vi "测量流程.vi"(11 "控制命令":T1(ring)) -> ()   [LabVIEW 2016, in "斯坦道CODcr.lvlib"]
uses:
  <vilib>/ptbypt/NI_PtbyPt.lvlib
panel:
  out "记录运行时间":timestamp
  out "start":timestamp
  out "重测":bool
  out "x-y":dbl
  out "当前时间":timestamp
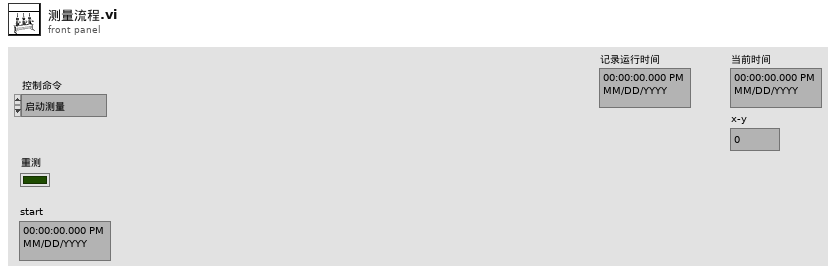
[diagram p1: front panel]
types:
  T1 = enum16{"启动测量", "标样核查", "零点核查", "跨度核查", "空白测试", "平行样测试", "加标回收", "空白校准", "标样校准", "初始化（清洗）", "停止测试", "仪器重启", "校时", "模式设置", "测量间隔设置"}
  T2 = cluster{"站号":u16, "量程切换":enum32{"H", "L", "AUTO"}, "控制命令":enum16{"启动测量", "标样核查", "零点核查", "跨度核查", "空白测试", "平行样测试", "加标回收", "空白校准", "标样校准", "初始化（清洗）", "停止测试", "仪器重启", "校时", "模式设置", "测量间隔设置"}, "模式设置":enum16{"待机", "连续模式", "周期模式", "定点模式", "受控模式", "手动模式"}, "测量间隔":u16}
  T3 = typedef "报警信息字段定义.ctl" = cluster{"时间":timestamp, "参数":string, "元器件":string, "故障现象":string, "故障分析":string, "state":string, "code":string, "platform_alarm_code":string}
  T4 = cluster{"时间标识":timestamp, "设备":string, "日志信息":string, "流程参数":string}
  T5 = enum16{"空闲", "水样测试", "标样核查", "零点核查", "跨度核查", "空白测试", "平行样测试", "加标回收", "空白校准", "标样校准", "初始化（清洗）"}
  T6 = cluster{"系统时间":timestamp, "工作状态":u16, "测量模式":enum16{"待机", "连续模式", "周期模式", "定点模式", "受控模式", "手动模式"}, "告警代码":u16, "故障代码":u16, "日志代码":u16, "软件版本":u16, "F0":sgl, "F1":sgl, "F2":sgl, "F3":sgl, "T":sgl, "H":sgl, "id":u16, "flowid":u16, "量程":u16, "总磷控温温度1":sgl, "营养盐控温温度2":sgl, "ADC":sgl}
  T7 = cluster{"水样测试量程模式":enum16{"H", "L", "AUTO"}, "空白核查量程模式":enum16{"H", "L", "AUTO"}, "跨度核查量程模式":enum16{"H", "L", "AUTO"}, "加标回收量程模式":enum16{"H", "L", "AUTO"}, "标样核查量程模式":enum16{"H", "L", "AUTO"}}
  T8 = cluster{"因子编码":u32, "单位":u16, "标样参考值":sgl, "水样数据时间":timestamp, "水样实测值":sgl, "水样数据标识":string, "标样数据时间":timestamp, "标样实测值":sgl, "标样数据标识":string, "空白数据时间":timestamp, "空白实测值":sgl, "空白数据标识":string, "零点核查数据时间":timestamp, "零点核查实测值":sgl, "零点核查数据标识":string, "跨度核查数据时间":timestamp, "跨度核查实测值":sgl, "跨度核查数据标识":string, "加标回收数据时间":timestamp, "加标回收实测值":sgl, "加标回收数据标识":string, "平行样数据时间":timestamp, "平行样实测值":sgl, "平行样数据标识":string, "F0":sgl, "F1":sgl, "F2":sgl, "F3":sgl, "F4":sgl, "F5":sgl, "F6":sgl, "F7":sgl, "温度":sgl, "湿度":sgl, "X值":sgl, "fidrange":u16, "X1值":sgl}[]
  T9 = cluster{"因子编码":u32, "单位":u16, "标样参考值":sgl, "水样数据时间":timestamp, "水样实测值":sgl, "水样数据标识":string, "标样数据时间":timestamp, "标样实测值":sgl, "标样数据标识":string, "空白数据时间":timestamp, "空白实测值":sgl, "空白数据标识":string, "零点核查数据时间":timestamp, "零点核查实测值":sgl, "零点核查数据标识":string, "跨度核查数据时间":timestamp, "跨度核查实测值":sgl, "跨度核查数据标识":string, "加标回收数据时间":timestamp, "加标回收实测值":sgl, "加标回收数据标识":string, "平行样数据时间":timestamp, "平行样实测值":sgl, "平行样数据标识":string, "F0":sgl, "F1":sgl, "F2":sgl, "F3":sgl, "F4":sgl, "F5":sgl, "F6":sgl, "F7":sgl, "温度":sgl, "湿度":sgl, "X值":sgl, "fidrange":u16, "X1值":sgl}
  T10 = cluster{"总磷跨度值":dbl, "总磷零点标准液浓度":dbl, "总磷跨度标准液浓度":dbl, "总磷标准液标准浓度":dbl, "总氮跨度值":dbl, "总氮零点标准液浓度":dbl, "总氮跨度标准液浓度":dbl, "总氮标准液标准浓度":dbl, "COD跨度值":dbl, "COD零点标准液浓度":dbl, "COD跨度标准液浓度":dbl, "COD标准液标准浓度":dbl, "氨氮跨度值":dbl, "氨氮零点标准液浓度":dbl, "氨氮跨度标准液浓度":dbl, "氨氮标准液标准浓度":dbl, "磷酸盐跨度值":dbl, "磷酸盐零点标准液浓度":dbl, "磷酸盐跨度标准液浓度":dbl, "磷酸盐标准液标准浓度":dbl, "硝氮跨度值":dbl, "硝氮零点标准液浓度":dbl, "硝氮跨度标准液浓度":dbl, "硝氮标准液标准浓度":dbl, "亚硝氮跨度值":dbl, "亚硝氮零点标准液浓度":dbl, "亚硝氮跨度标准液浓度":dbl, "亚硝氮标准液标准浓度":dbl, "硫化物跨度值":dbl, "硫化物零点标准液浓度":dbl, "硫化物跨度标准液浓度":dbl, "硫化物标准液标准浓度":dbl, "硅酸盐跨度值":dbl, "硅酸盐零点标准液浓度":dbl, "硅酸盐跨度标准液浓度":dbl, "硅酸盐标准液标准浓度":dbl, "总磷零点标准液偏差":dbl, "总磷跨度标准液偏差":dbl, "总磷标准液标准偏差":dbl, "总氮零点标准液偏差":dbl, "总氮跨度标准液偏差":dbl, "总氮标准液标准偏差":dbl, "COD零点标准液偏差":dbl, "COD跨度标准液偏差":dbl, "COD标准液标准偏差":dbl, "氨氮零点标准液偏差":dbl, "氨氮跨度标准液偏差":dbl, "氨氮标准液标准偏差":dbl, "磷酸盐零点标准液偏差":dbl, "磷酸盐跨度标准液偏差":dbl, "磷酸盐标准液标准偏差":dbl, "硝氮零点标准液偏差":dbl, "硝氮跨度标准液偏差":dbl, "硝氮标准液标准偏差":dbl, "亚硝氮零点标准液偏差":dbl, "亚硝氮跨度标准液偏差":dbl, "亚硝氮标准液标准偏差":dbl, "硫化物零点标准液偏差":dbl, "硫化物跨度标准液偏差":dbl, "硫化物标准液标准偏差":dbl, "硅酸盐零点标准液偏差":dbl, "硅酸盐跨度标准液偏差":dbl, "硅酸盐标准液标准偏差":dbl, "氟化物跨度值":dbl, "氟化物零点标准液浓度":dbl, "氟化物跨度标准液浓度":dbl, "氟化物标准液标准浓度":dbl, "氟化物零点标准液偏差":dbl, "氟化物跨度标准液偏差":dbl, "氟化物标准液标准偏差":dbl, "CODMn跨度值":dbl, "CODMn零点标准液浓度":dbl, "CODMn跨度标准液浓度":dbl, "CODMn标准液标准浓度":dbl, "CODMn零点标准液偏差":dbl, "CODMn跨度标准液偏差":dbl, "CODMn标准液标准偏差":dbl}
  T11 = typedef "LVDateTimeRec.ctl" = cluster{"秒数的小数部分":dbl, "秒":i32, "分":i32, "时":i32, "日":i32, "月":i32, "年":i32, "天数（周）":i32, "天数（年）":i32, "DST":i32}
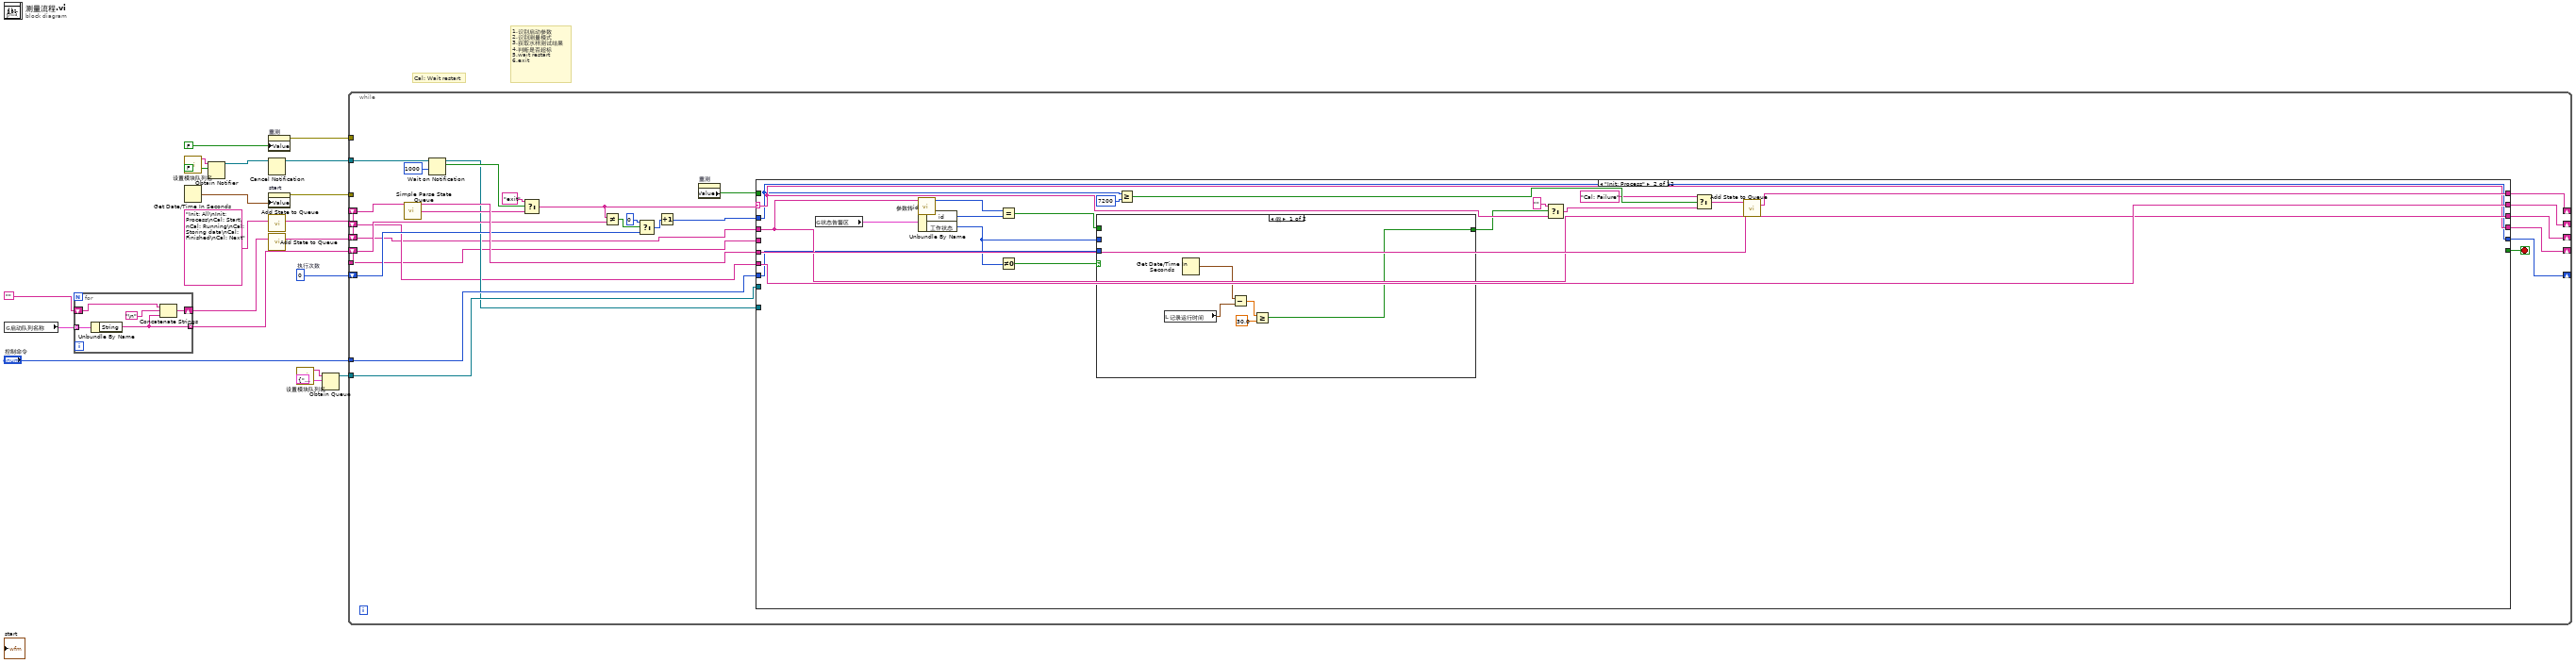
[diagram p0: block diagram]
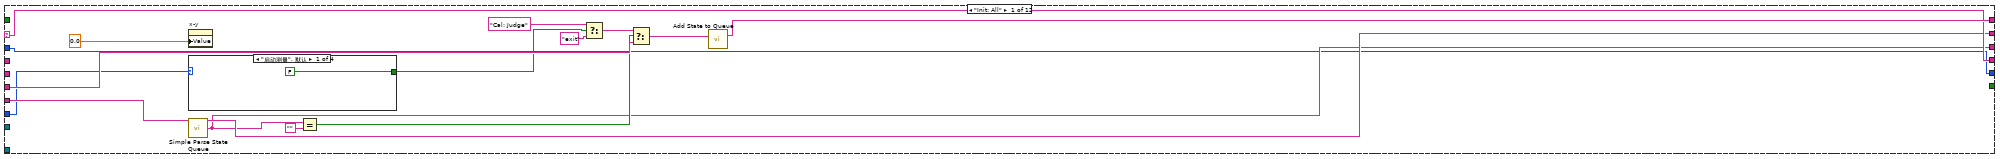
[diagram p2: hidden frame]
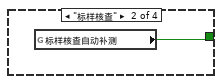
[diagram p3: hidden frame]
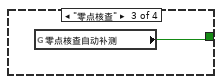
[diagram p4: hidden frame]
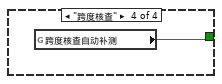
[diagram p5: hidden frame]
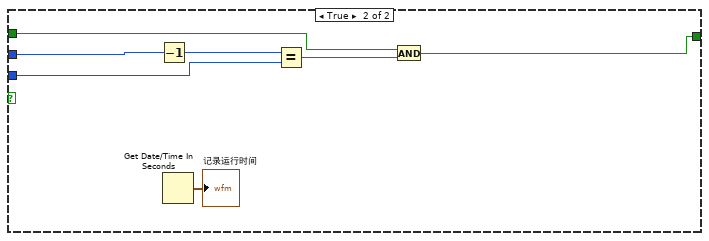
[diagram p6: hidden frame]
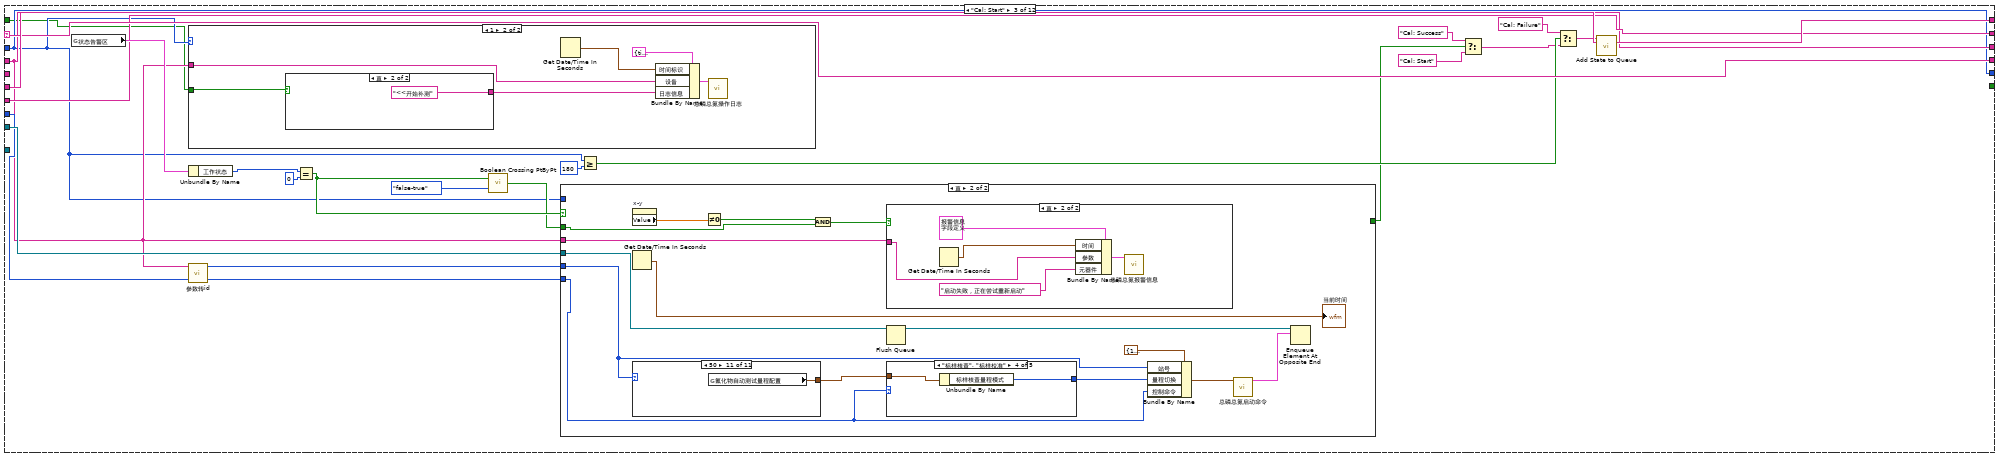
[diagram p7: hidden frame]
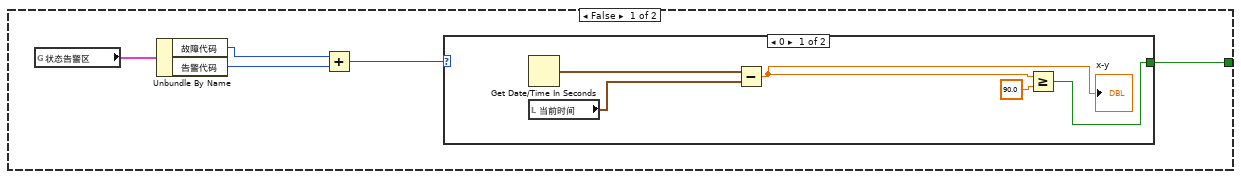
[diagram p8: hidden frame]
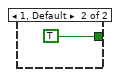
[diagram p9: hidden frame]
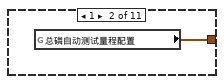
[diagram p12: hidden frame]
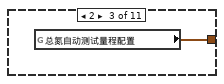
[diagram p13: hidden frame]
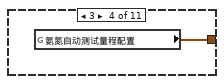
[diagram p14: hidden frame]
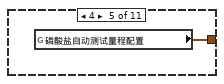
[diagram p15: hidden frame]
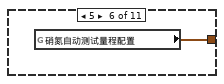
[diagram p16: hidden frame]
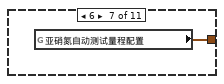
[diagram p17: hidden frame]
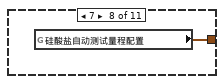
[diagram p18: hidden frame]
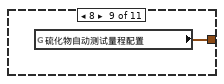
[diagram p19: hidden frame]
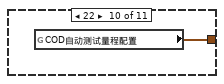
[diagram p20: hidden frame]
diagram:
  w14 = 0  # 执行次数
  # "Cal: Wait restart"
  # "1.识别启动参数\n2.识别测量模式\n3.获取水样测试结果\n4.判断是否超标\n5.wait restart\n6.exit"
  n1 = global read "model config var.vi" "启动队列名称"() -> (w7:cluster{"String":string, "Value":u16}[])
  n2 = for {
    shift-right: [w24] -> w8
    shift-left: "" -> [w25]
    tunnel: w7 -> [w23] mode=indexing
    tunnel: [w21] -> w1 mode=indexing
    n3 = Unbundle By Name(w23) -> ("String"=w21:string)
    n4 = Concatenate Strings(w25, "\n", w21) -> (w24:string)
  }
  n5 = call "设置模块队列名.vi"() -> ("Msg"=w12:string)  [unwired: 5 in]
  n6 = Get Date/Time In Seconds() -> (seconds since 1Jan1904=w2:timestamp)
  n7 = Obtain Notifier(name (unnamed)=w12, notification data type=FALSE) -> (notifier out=w19:refnum<notifier>)  [unwired: 2 in, 2 out]
  n8 = property on="重测" class="Bool (严格)"("Value"=FALSE ("重测")) -> (error out=w4:errorcluster)  [unwired: 2 in, 1 out]
  n9 = Cancel Notification(0:w19) -> (8:w10:refnum<notifier>)  [unwired: 1 in, 2 out]
  n10 = property on="start" class="AbsTime (严格)"("Value"=w2) -> (error out=w3:errorcluster)  [unwired: 2 in, 1 out]
  n11 = call "Add State to Queue.vi"("State(s) In (\"\")"="Init: All\nInit: Process\nCal: Start\nCal: Running\nCal: Storing data\nCal: Finished\nCal: Next" ("State(s) In (\"\")")) -> ("States Out"=w17:string)  [unwired: 14 in]
  n12 = call "Add State to Queue.vi"("State(s) In (\"\")"=w8) -> ("States Out"=w13:string)  [unwired: 14 in]
  n13 = call "设置模块队列名.vi"() -> ("Msg"=w11:string)  [unwired: 5 in]
  n14 = Obtain Queue(name (unnamed)=w11, element data type=cluster{"命令":string, "data":variant} {"命令"="", "data"=variant}) -> (queue out=w15:refnum<queue>)  [unwired: 3 in, 2 out]
  n15 = while {
    tunnel: w15 -> [w50]
    shift-right: [w49] -> _
    shift-left: w17 -> [w52]
    shift-right: [w43] -> _
    shift-left: w14 -> [w46]
    shift-right: [w27] -> _
    shift-left: _ -> [w48]
    tunnel: "控制命令" -> [w41]
    shift-right: [w39] -> _
    shift-left: w13 -> [w30]
    shift-right: [w28] -> _
    shift-left: _ -> [w29]
    tunnel: w10 -> [w37]
    tunnel: w4 -> [_]
    tunnel: w3 -> [_]
    tunnel: w1 -> [w26]
    stop <- w40 stop-if-true
    n16 = call "Simple Parse State Queue.vi"("State Queue"=w52) -> ("Remain States"=w51:string, "Next State"=w34:string)  [unwired: 13 in]
    n17 = Wait on Notification(notifier=w37, timeout in ms (-1)=1000 ("超时毫秒(-1)")) -> (notifier out=w32:refnum<notifier>, notification=w36:bool)  [unwired: 2 in, 2 out]
    n18 = Select(t="exit", s=w36, f=w34) -> (s? t:f=w33:string)
    n19 = Not Equal?(x=w33, y=w48) -> (x != y?=w47:bool)
    n20 = Select(t=0, s=w47, f=w46) -> (s? t:f=w44:i32)
    n21 = Increment(x=w44) -> (x+1=w42:i32)
    n22 = property on="重测" class="Bool (严格)"() -> ("Value"=w31:bool)  [unwired: 2 in, 2 out]
    n23 = case shown="\"Init: Process\"" w33 {
      selector: w33 -> [w67 w81 w126 w191 w206 w212 w226 w243 w260 w273 w437 w458]
      tunnel: w51 -> [w64 w91 w128 w193 _ w223 w231 w245 w257 _ _ w459]
      tunnel: w50 -> [_ _ w124 _ _ _ _ _ _ _ _ w455]
      tunnel: [w68 w92 w127 w192 w207 w222 w230 w244 w256 w261 w445 w459] -> w49
      tunnel: [w67 w81 w126 w191 w206 w212 w226 w243 w260 w273 w437 w458] -> w27
      tunnel: [w58 w80 w106 w190 w205 w215 w229 w241 w255 w274 w448 w457] -> w43
      tunnel: w42 -> [w58 w80 w106 w190 w205 w215 w229 w241 w255 w274 w448 w457]
      tunnel: w41 -> [w57 w85 w123 _ _ _ _ _ _ w272 _ _]
      tunnel: [_ _ _ _ _ _ _ _ _ _ _ TRUE] -> w40
      tunnel: w30 -> [w62 w90 w114 w189 w199 w209 w233 w242 w259 w267 w447 w456]
      tunnel: [w59 w88 w108 w188 w198 w208 w232 w240 w258 w269 w446 w453] -> w28
      tunnel: [w61 w90 w114 w189 w199 w209 w233 w242 w259 w266 w447 w456] -> w39
      tunnel: w29 -> [_ w88 w108 w188 w198 w208 w232 w240 w258 w269 w446 w453]
      tunnel: w32 -> [_ _ _ _ _ _ _ _ _ _ _ w454]
      tunnel: w31 -> [_ _ w105 _ _ _ _ w239 _ w271 _ _]
      tunnel: w26 -> [_ _ _ _ _ _ _ _ _ w268 _ _]
      frame "Init: All" {
        n24 = property on="x-y" class="DigNum (严格)"("Value"=0.0 ("x-y")) -> ()  [unwired: 2 in, 2 out]
        n25 = case shown="\"启动测量\", 默认" w57 {
          tunnel: [FALSE ("跨度核查自动补测") w70 w71 w72] -> w56
          frame "启动测量", Default {
          }
          frame "标样核查" {
            n26 = global read "总磷总氮断电保存全局变量.vi" "标样核查自动补测"() -> (w70:bool)
          }
          frame "零点核查" {
            n27 = global read "总磷总氮断电保存全局变量.vi" "零点核查自动补测"() -> (w71:bool)
          }
          frame "跨度核查" {
            n28 = global read "总磷总氮断电保存全局变量.vi" "跨度核查自动补测"() -> (w72:bool)
          }
        }
        n29 = call "Simple Parse State Queue.vi"("State Queue"=w62) -> ("Remain States"=w61:string, "Next State"=w59:string)  [unwired: 13 in]
        n30 = Equal?(x=w59, y="") -> (x = y?=w60:bool)
        n31 = Select(t="Cal: Judge", s=w56, f="exit") -> (s? t:f=w53:string)
        n32 = Select(t=w53, s=w60, f=w64) -> (s? t:f=w63:string)
        n33 = call "Add State to Queue.vi"("State(s) In (\"\")"=w63) -> ("States Out"=w68:string)  [unwired: 14 in]
      }
      frame "Init: Process" {
        n34 = global read "VAR总磷总氮全局变量.vi" "状态告警区"() -> (w89:T6)
        n35 = call "参数转id.vi"("table"=w88) -> ("id"=w86:u16)  [unwired: 10 in]
        n36 = Unbundle By Name(w89) -> ("id"=w87:u16, "工作状态"=w83:u16)
        n37 = Equal?(x=w86, y=w87) -> (x = y?=w74:bool)
        n38 = Not Equal To 0?(x=w83) -> (x != 0?=w84:bool)
        n39 = case shown="假" w84 {
          tunnel: w83 -> [_ w104]
          tunnel: w85 -> [_ w102]
          tunnel: [w93 w99] -> w73
          tunnel: w74 -> [_ w100]
          frame False {
            n40 = local read "记录运行时间"() -> (w97:timestamp)
            n41 = Get Date/Time In Seconds() -> (seconds since 1Jan1904=w96:timestamp)
            n42 = Subtract(x=w96, y=w97) -> (x-y=w95:dbl)
            n43 = Greater Or Equal?(x=w95, y=30.0) -> (x >= y?=w93:bool)
          }
          frame True {
            n44 = Decrement(x=w104) -> (x-1=w103:u16)
            n45 = Get Date/Time In Seconds() -> (seconds since 1Jan1904=→"记录运行时间":timestamp)
            n46 = Equal?(x=w103, y=w102) -> (x = y?=w101:bool)
            n47 = And(x=w100, y=w101) -> (x .and. y?=w99:bool)
          }
        }
        n48 = Greater Or Equal?(x=w80, y=7200) -> (x >= y?=w78:bool)
        n49 = Select(t="", s=w73, f=w81) -> (s? t:f=w76:string)
        n50 = Select(t="Cal: Failure", s=w78, f=w76) -> (s? t:f=w75:string)
        n51 = call "Add State to Queue.vi"("State(s) In Front (\"\")"=w75, "State(s) In (\"\")"=w91) -> ("States Out"=w92:string)  [unwired: 13 in]
      }
      frame "Cal: Start" {
        n52 = global read "VAR总磷总氮全局变量.vi" "状态告警区"() -> (w125:T6)
        n53 = case shown="1" w106 {
          tunnel: w108 -> [_ w181]
          tunnel: w105 -> [_ w180]
          frame 0, Default {
          }
          frame 1 {
            n54 = case shown="真" w180 {
              tunnel: ["<<开始测量" ("日志信息") "<<开始补测" ("日志信息")] -> w182
              frame False {
              }
              frame True {
              }
            }
            n55 = Get Date/Time In Seconds() -> (seconds since 1Jan1904=w185:timestamp)
            n56 = Bundle By Name(cluster=T4 {"时间标识"=timestamp(0 s since 1904-01-01), "设备"="", "日志信息"="", "流程参数"=""} ("data in"), "时间标识"=w185, "设备"=w181, "日志信息"=w182) -> (w184:T4)
            n57 = call "总磷总氮操作日志.vi"("data in"=w184) -> ()  [unwired: 10 in, 1 out]
          }
        }
        n58 = Unbundle By Name(w125) -> ("工作状态"=w113:u16)
        n59 = call "参数转id.vi"("table"=w108) -> ("id"=w107:u16)  [unwired: 10 in]
        n60 = Equal?(x=w113, y=u16 0) -> (x = y?=w111:bool)
        n61 = call <vilib>:"Boolean Crossing PtByPt.vi"("direction"=enum16{"either", "false-true", "true-false"}."false-true", "input"=w111) -> ("crossing"=w109:bool)  [unwired: 1 in]
        n62 = case shown="真" w111 {
          tunnel: w123 -> [_ w150]
          tunnel: w124 -> [_ w153]
          tunnel: [w133 _] -> w118
          tunnel: w107 -> [_ w148]
          tunnel: w106 -> [_ _]
          tunnel: w108 -> [_ w142]
          tunnel: w109 -> [_ w140]
          frame False {
            n63 = global read "VAR总磷总氮全局变量.vi" "状态告警区"() -> (w132:T6)
            n64 = Unbundle By Name(w132) -> ("故障代码"=w130:u16, "告警代码"=w131:u16)
            n65 = Add(x=w130, y=w131) -> (x+y=w129:u16)
            n66 = case shown="0" w129 {
              tunnel: [w134 TRUE] -> w133
              frame 0 {
                n67 = Get Date/Time In Seconds() -> (seconds since 1Jan1904=w137:timestamp)
                n68 = local read "当前时间"() -> (w138:timestamp)
                n69 = Subtract(x=w137, y=w138) -> (x-y=w136:dbl)
                "x-y" <- w136
                n70 = Greater Or Equal?(x=w136, y=90.0) -> (x >= y?=w134:bool)
              }
              frame 1, Default {
              }
            }
          }
          frame True {
            n71 = property on="x-y" class="DigNum (严格)"() -> ("Value"=w144:dbl)  [unwired: 2 in, 2 out]
            n72 = Get Date/Time In Seconds() -> (seconds since 1Jan1904=→"当前时间":timestamp)
            n73 = case shown="50" w148 {
              tunnel: [_ w160 w161 w162 w163 w164 w165 w166 w167 w168 w169] -> w149
              frame 0, Default {
              }
              frame 1 {
                n74 = global read "总磷总氮断电保存全局变量.vi" "总磷自动测试量程配置"() -> (w160:T7)
              }
              frame 2 {
                n75 = global read "总磷总氮断电保存全局变量.vi" "总氮自动测试量程配置"() -> (w161:T7)
              }
              frame 3 {
                n76 = global read "总磷总氮断电保存全局变量.vi" "氨氮自动测试量程配置"() -> (w162:T7)
              }
              frame 4 {
                n77 = global read "总磷总氮断电保存全局变量.vi" "磷酸盐自动测试量程配置"() -> (w163:T7)
              }
              frame 5 {
                n78 = global read "总磷总氮断电保存全局变量.vi" "硝氮自动测试量程配置"() -> (w164:T7)
              }
              frame 6 {
                n79 = global read "总磷总氮断电保存全局变量.vi" "亚硝氮自动测试量程配置"() -> (w165:T7)
              }
              frame 7 {
                n80 = global read "总磷总氮断电保存全局变量.vi" "硅酸盐自动测试量程配置"() -> (w166:T7)
              }
              frame 8 {
                n81 = global read "总磷总氮断电保存全局变量.vi" "硫化物自动测试量程配置"() -> (w167:T7)
              }
              frame 22 {
                n82 = global read "总磷总氮断电保存全局变量.vi" "COD自动测试量程配置"() -> (w168:T7)
              }
              frame 50 {
                n83 = global read "总磷总氮断电保存全局变量.vi" "氟化物自动测试量程配置"() -> (w169:T7)
              }
            }
            n84 = Not Equal To 0?(x=w144) -> (x != 0?=w143:bool)
            n85 = And(x=w143, y=w140) -> (x .and. y?=w141:bool)
            n86 = case shown="真" w141 {
              tunnel: w142 -> [_ w157]
              frame False {
              }
              frame True {
                n87 = Get Date/Time In Seconds() -> (seconds since 1Jan1904=w156:timestamp)
                n88 = Bundle By Name(cluster=T3 {"时间"=timestamp(0 s since 1904-01-01), "参数"="", "元器件"="", "故障现象"="", "故障分析"="", "state"="", "code"="", "platform_alarm_code"=""} ("data in"), "时间"=w156, "参数"=w157, "元器件"="启动失败，正在尝试重新启动" ("报警信息")) -> (w158:T3)
                n89 = call "总磷总氮报警信息.vi"("data in"=w158) -> ()  [unwired: 10 in, 1 out]
              }
            }
            n90 = Flush Queue(queue=w153) -> (queue out=w146:refnum<queue>)  [unwired: 1 in, 2 out]
            n91 = case shown="\"标样核查\", \"标样校准\"" w150 {
              tunnel: w149 -> [w171 w173 w175 w177 w179]
              tunnel: [w170 w172 w174 w176 w178] -> w154
              frame "启动测量", Default {
                n92 = Unbundle By Name(w171) -> ("水样测试量程模式"=w170:enum16{"H", "L", "AUTO"})
              }
              frame "零点核查", "空白测试", "空白校准" {
                n93 = Unbundle By Name(w173) -> ("空白核查量程模式"=w172:enum16{"H", "L", "AUTO"})
              }
              frame "跨度核查" {
                n94 = Unbundle By Name(w175) -> ("跨度核查量程模式"=w174:enum16{"H", "L", "AUTO"})
              }
              frame "标样核查", "标样校准" {
                n95 = Unbundle By Name(w177) -> ("标样核查量程模式"=w176:enum16{"H", "L", "AUTO"})
              }
              frame "加标回收" {
                n96 = Unbundle By Name(w179) -> ("加标回收量程模式"=w178:enum16{"H", "L", "AUTO"})
              }
            }
            n97 = Bundle By Name(cluster=T2 {"站号"=1, "量程切换"=enum."AUTO", "控制命令"=enum."启动测量", "模式设置"=enum."待机", "测量间隔"=0} ("参数"), "站号"=w148, "量程切换"=w154, "控制命令"=w150) -> (w151:T2)
            n98 = call "总磷总氮启动命令.vi"("参数"=w151) -> ("启动命令"=w147:cluster{"命令":string, "data":variant})  [unwired: 10 in]
            n99 = Enqueue Element At Opposite End(queue=w146, element=w147) -> ()  [unwired: 2 in, 3 out]
          }
        }
        n100 = Greater Or Equal?(x=w106, y=180) -> (x >= y?=w121:bool)
        n101 = Select(t="Cal: Success" ("State(s) In (\"\")"), s=w118, f="Cal: Start" ("State(s) In (\"\")")) -> (s? t:f=w116:string)
        n102 = Select(t="Cal: Failure" ("State(s) In (\"\")"), s=w121, f=w116) -> (s? t:f=w119:string)
        n103 = call "Add State to Queue.vi"("State(s) In Front (\"\")"=w119, "State(s) In (\"\")"=w128) -> ("States Out"=w127:string)  [unwired: 13 in]
      }
      frame "Cal: Success" {
        n104 = Get Date/Time In Seconds() -> (seconds since 1Jan1904=w196:timestamp)
        n105 = Bundle By Name(cluster=T4 {"时间标识"=timestamp(0 s since 1904-01-01), "设备"="", "日志信息"="", "流程参数"=""} ("data in"), "时间标识"=w196, "设备"=w188, "日志信息"="启动成功") -> (w195:T4)
        n106 = call "总磷总氮操作日志.vi"("data in"=w195) -> ()  [unwired: 10 in, 1 out]
        n107 = call "Add State to Queue.vi"("State(s) In (\"\")"=w193) -> ("States Out"=w192:string)  [unwired: 14 in]
      }
      frame "Cal: Failure" {
        n108 = Get Date/Time In Seconds() -> (seconds since 1Jan1904=w203:timestamp)
        n109 = Bundle By Name(cluster=T4 {"时间标识"=timestamp(0 s since 1904-01-01), "设备"="", "日志信息"="", "流程参数"=""} ("data in"), "时间标识"=w203, "设备"=w198, "日志信息"="启动失败") -> (w202:T4)
        n110 = call "总磷总氮操作日志.vi"("data in"=w202) -> ()  [unwired: 10 in, 1 out]
        n111 = call "Add State to Queue.vi"("State(s) In (\"\")"="exit" ("State(s) In (\"\")")) -> ("States Out"=w207:string)  [unwired: 14 in]
      }
      frame "Cal: Running" {
        n112 = global read "VAR总磷总氮全局变量.vi" "状态告警区"() -> (w219:T6)
        n113 = Unbundle By Name(w219) -> ("工作状态"=w220:u16)
        n114 = Less Or Equal?(x=w215, y=7200) -> (x <= y?=w213:bool)
        n115 = Select(t=w212, s=w213, f="exit") -> (s? t:f=w211:string)
        n116 = Equal?(x=w220, y=T5."空闲") -> (x = y?=w218:bool)
        n117 = Select(t="", s=w218, f=w211) -> (s? t:f=w216:string)
        n118 = call "Add State to Queue.vi"("State(s) In Front (\"\")"=w216, "State(s) In (\"\")"=w223) -> ("States Out"=w222:string)  [unwired: 13 in]
      }
      frame "Cal: Storing data" {
        n119 = case shown="1" w229 {
          tunnel: w232 -> [_ w234]
          frame 0, Default {
          }
          frame 1 {
            n120 = Get Date/Time In Seconds() -> (seconds since 1Jan1904=w238:timestamp)
            n121 = Bundle By Name(cluster=T4 {"时间标识"=timestamp(0 s since 1904-01-01), "设备"="", "日志信息"="", "流程参数"=""} ("data in"), "时间标识"=w238, "设备"=w234, "日志信息"="存储数据") -> (w237:T4)
            n122 = call "总磷总氮操作日志.vi"("data in"=w237) -> ()  [unwired: 10 in, 1 out]
          }
        }
        n123 = Less Or Equal?(x=w229, y=60) -> (x <= y?=w227:bool)
        n124 = Select(t=w226, s=w227, f="") -> (s? t:f=w224:string)
        n125 = call "Add State to Queue.vi"("State(s) In Front (\"\")"=w224, "State(s) In (\"\")"=w231) -> ("States Out"=w230:string)  [unwired: 13 in]
      }
      frame "Cal: Finished" {
        n126 = case shown="1" w241 {
          tunnel: w240 -> [_ w247]
          tunnel: w239 -> [_ w246]
          frame 0, Default {
          }
          frame 1 {
            n127 = case shown="假" w246 {
              tunnel: ["测量结束>>" ("日志信息") "补测结束>>" ("日志信息")] -> w248
              frame False {
              }
              frame True {
              }
            }
            n128 = Get Date/Time In Seconds() -> (seconds since 1Jan1904=w251:timestamp)
            n129 = Bundle By Name(cluster=T4 {"时间标识"=timestamp(0 s since 1904-01-01), "设备"="", "日志信息"="", "流程参数"=""} ("data in"), "时间标识"=w251, "设备"=w247, "日志信息"=w248) -> (w250:T4)
            n130 = call "总磷总氮操作日志.vi"("data in"=w250) -> ()  [unwired: 10 in, 1 out]
          }
        }
        n131 = call "Add State to Queue.vi"("State(s) In (\"\")"=w245) -> ("States Out"=w244:string)  [unwired: 14 in]
      }
      frame "Cal: Next" {
        n132 = call "Add State to Queue.vi"("State(s) In Front (\"\")"="Init: All\nInit: Process\nCal: Start\nCal: Running\nCal: Storing data\nCal: Finished\nCal: Next" ("State(s) In (\"\")"), "State(s) In (\"\")"=w257) -> ("States Out"=w256:string)  [unwired: 13 in]
      }
      frame "Cal: Judge" {
        n133 = Not(x=w271) -> (.not. x?=w270:bool)
        n134 = for {
          tunnel: w272 -> [w281]
          tunnel: w270 -> [w280]
          tunnel: w268 -> [w279] mode=indexing
          shift-right: [w277] -> w266
          shift-left: w267 -> [w278]
          shift-right: [w276] -> w264
          shift-left: FALSE -> [w275]
          n135 = case shown="真" w280 {
            tunnel: w281 -> [_ w295]
            tunnel: w279 -> [_ w288]
            tunnel: w278 -> [_ w287]
            tunnel: ["" ("States Out") w286] -> w277
            tunnel: [FALSE w285] -> w276
            tunnel: w275 -> [_ w284]
            frame False {
              # "继续测试下一个参数/EXIT"
            }
            frame True {
              # "参数测完-判定是否超标"
              n136 = call "参数转id.vi"("table"=w288) -> ("id"=w289:u16)  [unwired: 10 in]
              n137 = call "id参数转换.vi"("id"=w289) -> ("数组资源索引"=w294:i32)  [unwired: 9 in, 1 out]
              n138 = global read "VAR总磷总氮全局变量.vi" "测量数据区数组"() -> (w293:T8)
              n139 = Index Array(array=w293, index=w294) -> (element=w292:T9)
              n140 = case shown="\"跨度核查\"" w295 {
                tunnel: w292 -> [_ w314 w365 w405]
                tunnel: w289 -> [_ w312 w366 w404]
                tunnel: [TRUE w310 w363 w402] -> w291
                tunnel: [_ "标样核查不合格" ("日志信息") "零点核查不合格" ("日志信息") "跨度核查不合格" ("日志信息")] -> w290
                frame "启动测量", Default {
                }
                frame "标样核查" {
                  n141 = global read "总磷总氮断电保存全局变量.vi" "质控参数设置"() -> (w313:T10)
                  n142 = Unbundle By Name(w314) -> ("标样实测值"=w307:sgl)
                  n143 = case shown="5" w312 {
                    tunnel: w313 -> [_ w317 w320 w323 w326 w329 w332 w339 w346 w353 w360]
                    tunnel: [_ w316 w319 w322 w325 w328 w331 w338 w345 w352 w359] -> w309
                    tunnel: [_ w315 w318 w321 w324 w327 w330 w337 w344 w351 w358] -> w308
                    frame Default {
                    }
                    frame 1 {
                      n144 = Unbundle By Name(w317) -> ("总磷标准液标准浓度"=w316:dbl, "总磷标准液标准偏差"=w315:dbl)
                    }
                    frame 2 {
                      n145 = Unbundle By Name(w320) -> ("总氮标准液标准浓度"=w319:dbl, "总氮标准液标准偏差"=w318:dbl)
                    }
                    frame 3 {
                      n146 = Unbundle By Name(w323) -> ("氨氮标准液标准浓度"=w322:dbl, "氨氮标准液标准偏差"=w321:dbl)
                    }
                    frame 4 {
                      n147 = Unbundle By Name(w326) -> ("磷酸盐标准液标准浓度"=w325:dbl, "磷酸盐标准液标准偏差"=w324:dbl)
                    }
                    frame 5 {
                      n148 = Unbundle By Name(w329) -> ("硝氮标准液标准浓度"=w328:dbl, "硝氮标准液标准偏差"=w327:dbl)
                    }
                    frame 6 {
                      n149 = Unbundle By Name(w332) -> ("亚硝氮标准液标准浓度"=w334:dbl, "亚硝氮标准液标准偏差"=w336:dbl)
                      n150 = Multiply(x=w336, y=0.01) -> (x*y=w333:dbl)
                      n151 = Add(x=w334, y=w333) -> (x+y=w331:dbl)
                      n152 = Subtract(x=w334, y=w333) -> (x-y=w330:dbl)
                    }
                    frame 7 {
                      n153 = Unbundle By Name(w339) -> ("硅酸盐标准液标准浓度"=w341:dbl, "硅酸盐标准液标准偏差"=w343:dbl)
                      n154 = Multiply(x=w343, y=0.01) -> (x*y=w340:dbl)
                      n155 = Add(x=w341, y=w340) -> (x+y=w338:dbl)
                      n156 = Subtract(x=w341, y=w340) -> (x-y=w337:dbl)
                    }
                    frame 8 {
                      n157 = Unbundle By Name(w346) -> ("硫化物标准液标准浓度"=w348:dbl, "硫化物标准液标准偏差"=w350:dbl)
                      n158 = Multiply(x=w350, y=0.01) -> (x*y=w347:dbl)
                      n159 = Add(x=w348, y=w347) -> (x+y=w345:dbl)
                      n160 = Subtract(x=w348, y=w347) -> (x-y=w344:dbl)
                    }
                    frame 22 {
                      n161 = Unbundle By Name(w353) -> ("COD标准液标准浓度"=w355:dbl, "COD标准液标准偏差"=w357:dbl)
                      n162 = Multiply(x=w357, y=0.01) -> (x*y=w354:dbl)
                      n163 = Add(x=w355, y=w354) -> (x+y=w352:dbl)
                      n164 = Subtract(x=w355, y=w354) -> (x-y=w351:dbl)
                    }
                    frame 50 {
                      n165 = Unbundle By Name(w360) -> ("氟化物标准液标准浓度"=w359:dbl, "氟化物标准液标准偏差"=w358:dbl)
                    }
                  }
                  n166 = call "相对标准偏差判断.vi"("实测值"=w307, "相对标准偏差"=w308, "标样值"=w309) -> ("合格？"=w310:bool)  [unwired: 8 in]
                }
                frame "零点核查" {
                  n167 = global read "总磷总氮断电保存全局变量.vi" "质控参数设置"() -> (w368:T10)
                  n168 = Unbundle By Name(w365) -> ("零点核查实测值"=w361:sgl)
                  n169 = case shown="3" w366 {
                    tunnel: w368 -> [_ w371 w374 w377 w380 w383 w386 w389 w392 w395 w398]
                    tunnel: [_ w370 w373 w376 w379 w382 w385 w388 w391 w394 w397] -> w367
                    tunnel: [_ w369 w372 w375 w378 w381 w384 w387 w390 w393 w396] -> w362
                    frame Default {
                    }
                    frame 1 {
                      n170 = Unbundle By Name(w371) -> ("总磷零点标准液浓度"=w370:dbl, "总磷零点标准液偏差"=w369:dbl)
                    }
                    frame 2 {
                      n171 = Unbundle By Name(w374) -> ("总氮零点标准液浓度"=w373:dbl, "总氮零点标准液偏差"=w372:dbl)
                    }
                    frame 3 {
                      n172 = Unbundle By Name(w377) -> ("氨氮零点标准液浓度"=w376:dbl, "氨氮零点标准液偏差"=w375:dbl)
                    }
                    frame 4 {
                      n173 = Unbundle By Name(w380) -> ("磷酸盐零点标准液浓度"=w379:dbl, "磷酸盐零点标准液偏差"=w378:dbl)
                    }
                    frame 5 {
                      n174 = Unbundle By Name(w383) -> ("硝氮零点标准液浓度"=w382:dbl, "硝氮零点标准液偏差"=w381:dbl)
                    }
                    frame 6 {
                      n175 = Unbundle By Name(w386) -> ("亚硝氮零点标准液浓度"=w385:dbl, "亚硝氮零点标准液偏差"=w384:dbl)
                    }
                    frame 7 {
                      n176 = Unbundle By Name(w389) -> ("硅酸盐零点标准液浓度"=w388:dbl, "硅酸盐零点标准液偏差"=w387:dbl)
                    }
                    frame 8 {
                      n177 = Unbundle By Name(w392) -> ("硫化物零点标准液浓度"=w391:dbl, "硫化物零点标准液偏差"=w390:dbl)
                    }
                    frame 22 {
                      n178 = Unbundle By Name(w395) -> ("COD零点标准液浓度"=w394:dbl, "COD零点标准液偏差"=w393:dbl)
                    }
                    frame 50 {
                      n179 = Unbundle By Name(w398) -> ("氟化物零点标准液浓度"=w397:dbl, "氟化物零点标准液偏差"=w396:dbl)
                    }
                  }
                  n180 = call "绝对标准偏差判断.vi"("实测值"=w361, "绝对标准偏差"=w362, "标准值"=w367) -> ("合格？"=w363:bool)  [unwired: 8 in]
                }
                frame "跨度核查" {
                  n181 = global read "总磷总氮断电保存全局变量.vi" "质控参数设置"() -> (w406:T10)
                  n182 = Unbundle By Name(w405) -> ("跨度核查实测值"=w401:sgl)
                  n183 = case shown="1" w404 {
                    tunnel: w406 -> [_ w409 w412 w415 w418 w421 w424 w427 w430 w433 w436]
                    tunnel: [_ w408 w411 w414 w417 w420 w423 w426 w429 w432 w435] -> w400
                    tunnel: [_ w407 w410 w413 w416 w419 w422 w425 w428 w431 w434] -> w399
                    frame Default {
                    }
                    frame 1 {
                      n184 = Unbundle By Name(w409) -> ("总磷跨度标准液浓度"=w408:dbl, "总磷跨度标准液偏差"=w407:dbl)
                    }
                    frame 2 {
                      n185 = Unbundle By Name(w412) -> ("总氮跨度标准液浓度"=w411:dbl, "总氮跨度标准液偏差"=w410:dbl)
                    }
                    frame 3 {
                      n186 = Unbundle By Name(w415) -> ("氨氮跨度标准液浓度"=w414:dbl, "氨氮跨度标准液偏差"=w413:dbl)
                    }
                    frame 4 {
                      n187 = Unbundle By Name(w418) -> ("磷酸盐跨度标准液浓度"=w417:dbl, "磷酸盐跨度标准液偏差"=w416:dbl)
                    }
                    frame 5 {
                      n188 = Unbundle By Name(w421) -> ("硝氮跨度标准液浓度"=w420:dbl, "硝氮跨度标准液偏差"=w419:dbl)
                    }
                    frame 6 {
                      n189 = Unbundle By Name(w424) -> ("亚硝氮跨度标准液浓度"=w423:dbl, "亚硝氮跨度标准液偏差"=w422:dbl)
                    }
                    frame 7 {
                      n190 = Unbundle By Name(w427) -> ("硅酸盐跨度标准液浓度"=w426:dbl, "硅酸盐跨度标准液偏差"=w425:dbl)
                    }
                    frame 8 {
                      n191 = Unbundle By Name(w430) -> ("硫化物跨度标准液浓度"=w429:dbl, "硫化物跨度标准液偏差"=w428:dbl)
                    }
                    frame 22 {
                      n192 = Unbundle By Name(w433) -> ("COD跨度标准液浓度"=w432:dbl, "COD跨度标准液偏差"=w431:dbl)
                    }
                    frame 50 {
                      n193 = Unbundle By Name(w436) -> ("氟化物跨度标准液浓度"=w435:dbl, "氟化物跨度标准液偏差"=w434:dbl)
                    }
                  }
                  n194 = call "相对标准偏差判断.vi"("实测值"=w401, "相对标准偏差"=w399, "标样值"=w400) -> ("合格？"=w402:bool)  [unwired: 8 in]
                }
              }
              n195 = case shown="假" w291 {
                tunnel: w288 -> [w297 _]
                tunnel: w290 -> [w300 _]
                tunnel: w287 -> [w299 w305]
                tunnel: [w298 w305] -> w286
                tunnel: [TRUE w304] -> w285
                tunnel: w284 -> [_ w304]
                frame False {
                  n196 = Get Date/Time In Seconds() -> (seconds since 1Jan1904=w303:timestamp)
                  n197 = call "Add State to Queue.vi"("State(s) In (\"\")"=w299, "State(s) At Back (\"\")"=w297) -> ("States Out"=w298:string)  [unwired: 13 in]
                  n198 = Bundle By Name(cluster=T4 {"时间标识"=timestamp(0 s since 1904-01-01), "设备"="", "日志信息"="", "流程参数"=""} ("data in"), "时间标识"=w303, "设备"=w297, "日志信息"=w300) -> (w302:T4)
                  n199 = call "总磷总氮操作日志.vi"("data in"=w302) -> ()  [unwired: 10 in, 1 out]
                }
                frame True {
                }
              }
            }
          }
        }
        n200 = Select(t="Cal: Wait restart" ("State(s) In (\"\")"), s=w264, f="exit" ("State(s) In (\"\")")) -> (s? t:f=w261:string)
      }
      frame "Cal: Wait restart" {
        n201 = local read "start"() -> (w444:timestamp)
        n202 = Get Date/Time In Seconds() -> (seconds since 1Jan1904=w441:timestamp)
        n203 = Seconds To Date/Time(time stamp (now)=w444) -> (date time rec=w443:T11)  [unwired: 1 in]
        n204 = Seconds To Date/Time(time stamp (now)=w441) -> (date time rec=w442:T11)  [unwired: 1 in]
        n205 = Unbundle By Name(w443) -> ("时"=w439:i32)
        n206 = Unbundle By Name(w442) -> ("时"=w440:i32)
        n207 = Not Equal?(x=w439, y=w440) -> (x != y?=w438:bool)
        n208 = case shown="真" w438 {
          tunnel: [w449 "Init: All\nInit: Process\nCal: Start\nCal: Running\nCal: Storing data\nCal: Finished\nCal: Next" ("State(s) In (\"\")")] -> w445
          tunnel: w437 -> [w449 _]
          frame False {
          }
          frame True {
            "重测" <- TRUE ("重测")
          }
        }
      }
      frame "exit", Default {
        n209 = Release Notifier(notifier=w454) -> ()  [unwired: 2 in, 3 out]
        n210 = Release Queue(queue=w455) -> ()  [unwired: 2 in, 3 out]
        n211 = Empty String/Path?(string/path=w453) -> (empty?=w452:bool)
        n212 = case shown="假" w452 {
          tunnel: w453 -> [w461 _]
          frame False {
            n213 = Get Date/Time In Seconds() -> (seconds since 1Jan1904=w465:timestamp)
            n214 = Bundle By Name(cluster=T4 {"时间标识"=timestamp(0 s since 1904-01-01), "设备"="", "日志信息"="", "流程参数"=""} ("data in"), "时间标识"=w465, "设备"=w461, "日志信息"="流程结束>>") -> (w464:T4)
            n215 = call "总磷总氮操作日志.vi"("data in"=w464) -> ()  [unwired: 10 in, 1 out]
          }
          frame True {
          }
        }
      }
    }
  }
